vi "VCI Open Device.vi"(9 "Reserved":u32, 10 "DevIndex":u32, 11 "DevType":u32) -> (3 "function return":u32)   [LabVIEW 2010, in "ControlCAN.lvlib"]
doc: "unsigned int WINAPI VCI_OpenDevice(unsigned int DevType,unsigned int DevIndex,unsigned int Reserved);"
uses:
  ControlCAN.lvlib
  ControlCAN/Ginkgo_Driver.dll
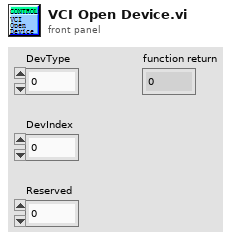
[diagram p1: front panel]
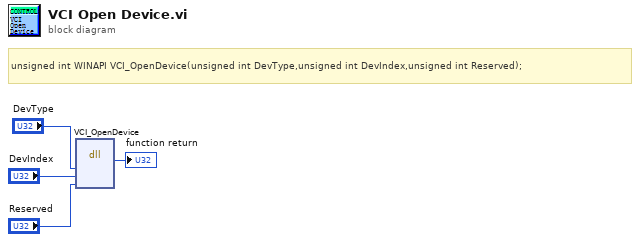
[diagram p0: block diagram]
diagram:
  # "unsigned int WINAPI VCI_OpenDevice(unsigned int DevType,unsigned int DevIndex,unsigned int Reserved);"
  n1 = dll-call lib="E:/Project/vt_ginkgo/truck/Ginkgo Driver/vs2010/Ginkgo_USB-I2C&SPI&CAN_API_v2.0.3.3/lib/labview_32bit/ControlCAN/Ginkgo_Driver.*" fn="VCI_OpenDevice"("DevType"="DevType", "DevIndex"="DevIndex", "Reserved"="Reserved") -> (→"function return":u32)  [unwired: 6 in, 2 out]
